vi "ATF Storage-DO waveform Samples bulider.vi"(9 "Data input":waveform(dbl)[](array[waveform])=[{"t0"=timestamp(3812260595.132041 s since 1904-01-01), "dt"=0.001, "Y"=[1.0, 1.0, 1.0, 1.0, 1.0], "attributes"=variant("NI_LineName"=variant(string "NO_EPV_1102"))}, {"t0"=timestamp(3812260595.132041 s since 1904-01-01), "dt"=0.001, "Y"=[0.0, 0.0, 0.0, 0.0, 0.0], "attributes"=variant("NI_LineName"=variant(string "NC_EPV_1214"))}, {"t0"=timestamp(3812260595.132041 s since 1904-01-01), "dt"=0.001, "Y"=[1.0, 1.0, 1.0, 1.0, 1.0], "attributes"=variant("NI_LineName"=variant(string "NO_EPV_1207"))}, {"t0"=timestamp(3812260595.132041 s since 1904-01-01), "dt"=0.001, "Y"=[0.0, 0.0, 0.0, 0.0, 0.0], "attributes"=variant("NI_LineName"=variant(string "AC_Button"))}, {"t0"=timestamp(3812260595.132041 s since 1904-01-01), "dt"=0.001, "Y"=[0.0, 0.0, 0.0, 0.0, 0.0], "attributes"=variant("NI_LineName"=variant(string "NC_EPV_1211"))}], 11 "DO_Data RD":refnum<queue>) -> ()   [LabVIEW 2022 SP3]
panel:
  out "x-y":u32
  out "overflow? 2":bool
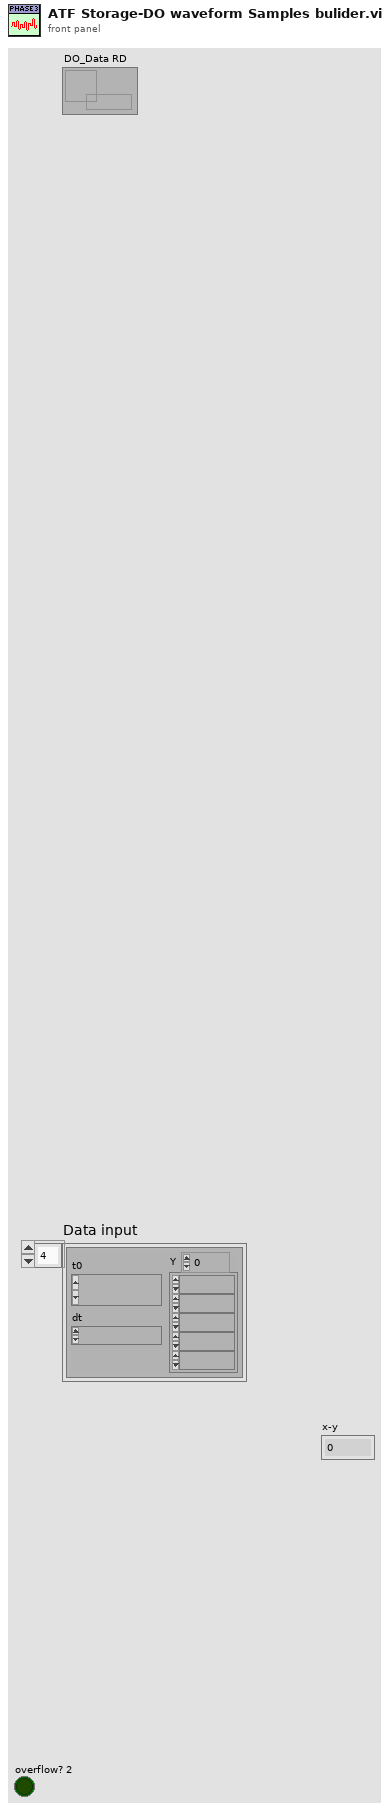
[diagram p1: front panel]
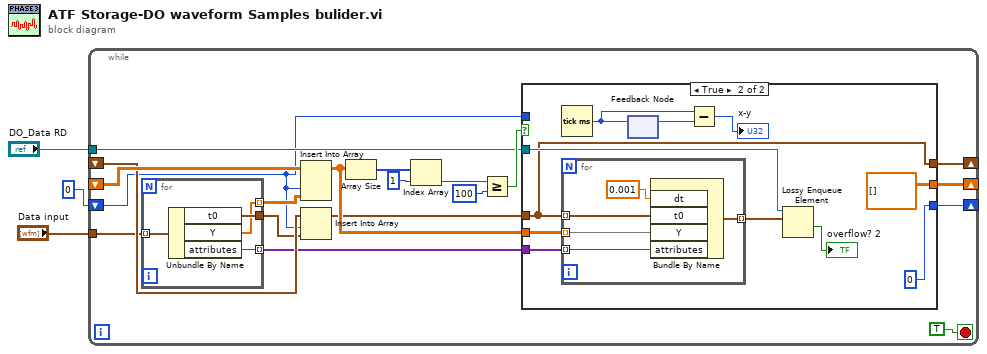
[diagram p0: block diagram]
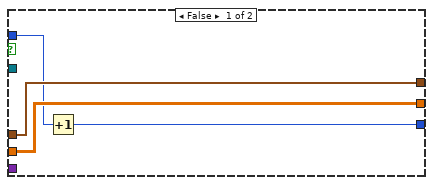
[diagram p2: hidden frame]
diagram:
  n1 = while {
    tunnel: "Data input" -> [w5]
    shift-right: [w18] -> _
    shift-left: _ -> [w22]
    shift-right: [w8] -> _
    shift-left: _ -> [w20]
    tunnel: "DO_Data RD" -> [w9]
    shift-right: [w7] -> _
    shift-left: 0 -> [w6]
    stop <- TRUE stop-if-true
    n2 = for {
      tunnel: w5 -> [w46] mode=indexing
      tunnel: [w43] -> w21 mode=indexing
      tunnel: [w45] -> w19
      tunnel: [w44] -> w10 mode=indexing
      n3 = Unbundle By Name(w46) -> ("t0"=w45:timestamp, "Y"=w43:dbl[], "attributes"=w44:variant)
    }
    n4 = Insert Into Array(array=w22, index (col)=w6, new element=w21) -> (w16:dbl[][])  [unwired: 1 in]
    n5 = Insert Into Array(array=w20, index=w6, new element=w19) -> (w11:timestamp[])
    n6 = Array Size(array=w16) -> (size(s)=w17:i32[])
    n7 = Index Array(array=w17, index=1) -> (element=w15:i32)
    n8 = Greater Or Equal?(x=w15, y=100) -> (x >= y?=w13:bool)
    n9 = case shown="True" w13 {
      tunnel: w16 -> [w26 w36]
      tunnel: [w26 dbl[][] []] -> w18
      tunnel: w11 -> [w25 w31]
      tunnel: w10 -> [_ w35]
      tunnel: w9 -> [_ w34]
      tunnel: [w25 w31] -> w8
      tunnel: w6 -> [w24 _]
      tunnel: [w23 0] -> w7
      frame False {
        n10 = Increment(x=w24) -> (x+1=w23:i32)
      }
      frame True {
        n11 = Tick Count (ms)() -> (millisecond timer value=w30:u32)
        n12 = for {
          tunnel: w36 -> [w42] mode=indexing
          tunnel: w31 -> [w41] mode=indexing
          tunnel: w35 -> [w40] mode=indexing
          tunnel: [w38] -> w33 mode=indexing
          n13 = Bundle By Name("dt"=0.001, "t0"=w41, "Y"=w42, "attributes"=w40) -> (w38:waveform(dbl))  [unwired: 1 in]
        }
        n14 = feedback #1() -> (w29:u32)  [unwired: 1 in]
        n15 = feedback-in #1(w30) -> ()
        n16 = Subtract(x=w30, y=w29) -> (x-y=→"x-y":u32)
        n17 = Lossy Enqueue Element(queue=w34, element=w33) -> (overflow?=→"overflow? 2":bool)  [unwired: 1 in, 3 out]
      }
    }
  }
